vi "util_timer.vi"(7 "timer_command":T2=enum."read", 8 "error in (no error)":errorcluster, 10 "current_time":dbl=nan format="%#_13g", 11 "timer in":T1 {"previous_time" format="%<%H:%M:%S%3u>t"; "elapsed_time" format="%<%H:%M:%S%3u>t"}) -> (0 "error out":errorcluster, 2 "elapsed_time":dbl format="%#_13g", 3 "timer out":T1 {"previous_time" format="%<%H:%M:%S%3u>t"; "elapsed_time" format="%<%H:%M:%S%3u>t"})   [LabVIEW 2015, in "lv-recipe-machine.lvlib"]
uses:
  lv-recipe-machine.lvlib
  _controls/timer_command.ctl
  public/_controls/timer.ctl
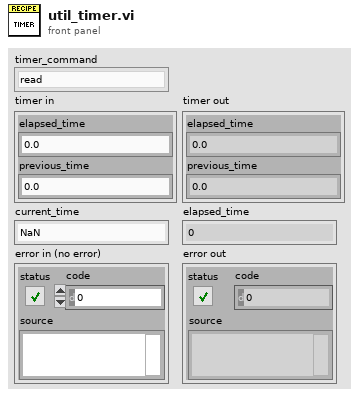
[diagram p1: front panel]
types:
  T1 = typedef "lv-recipe-machine.lvlib/timer.ctl" = cluster{"elapsed_time":dbl, "previous_time":dbl}
  T2 = typedef "lv-recipe-machine.lvlib/timer_command.ctl" = enum16{"<timer_command>", "start", "read", "pause", "resume", "stop", "<null>"}
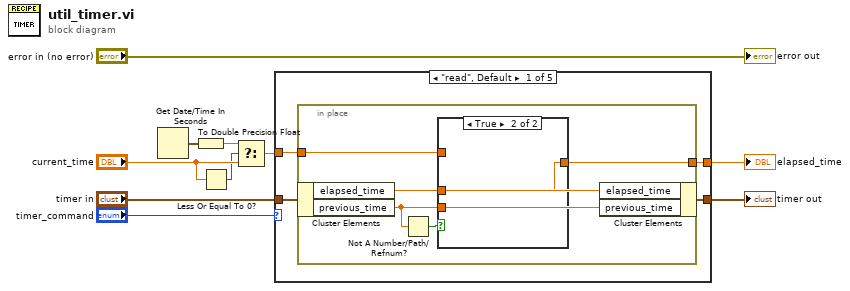
[diagram p0: block diagram]
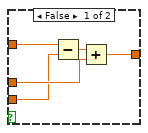
[diagram p2: hidden frame]
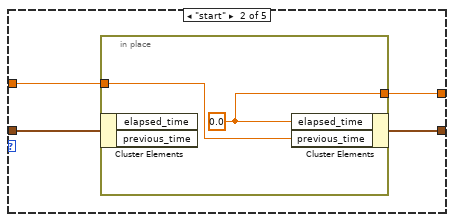
[diagram p3: hidden frame]
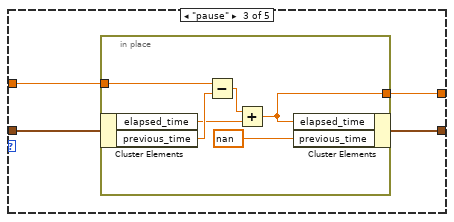
[diagram p4: hidden frame]
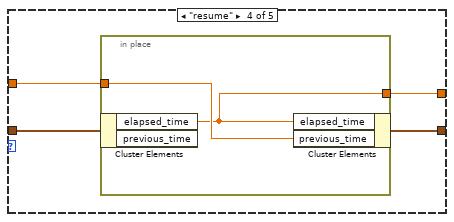
[diagram p5: hidden frame]
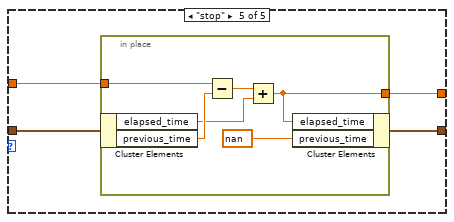
[diagram p6: hidden frame]
diagram:
  n1 = Get Date/Time In Seconds() -> (seconds since 1Jan1904=w3:timestamp)
  n2 = To Double Precision Float(number=w3) -> (double precision float=w2:dbl)
  n3 = Less Or Equal To 0?(x="current_time") -> (x <= 0?=w4:bool)
  n4 = Select(t=w2, s=w4, f="current_time") -> (s? t:f=w1:dbl)
  n5 = case shown="\"read\", Default" "timer_command" {
    tunnel: "timer in" -> [w14 w29 w35 w45 w51]
    tunnel: w1 -> [w13 w28 w34 w44 w50]
    tunnel: [w12 w27 w33 w43 w49] -> w6
    tunnel: [w11 w26 w32 w42 w48] -> w5
    frame "read", Default {
      n6 = in-place {
        in-place-border: w13 -> [w19]
        in-place-border: [w17] -> w11
        n7 = in-place-cluster #1(w14) -> ("elapsed_time"=w18:dbl, "previous_time"=w16:dbl)
        n8 = Not A Number/Path/Refnum?(number/path/refnum=w16) -> (NaN/Path/Refnum?=w15:bool)
        n9 = case shown="True" w15 {
          tunnel: w19 -> [w24 _]
          tunnel: w18 -> [w23 w25]
          tunnel: w16 -> [w22 _]
          tunnel: [w20 w25] -> w17
          frame False {
            n10 = Subtract(x=w24, y=w22) -> (x-y=w21:dbl)
            n11 = Add(x=w21, y=w23) -> (x+y=w20:dbl)
          }
          frame True {
          }
        }
        n12 = in-place-cluster #1("elapsed_time"=w18, "previous_time"=w16) -> (w12:T1)
      }
    }
    frame "start" {
      n13 = in-place {
        in-place-border: w28 -> [w31]
        in-place-border: [w30] -> w26
        w30 = 0.0 ("elapsed_timer")
        n14 = in-place-cluster #2(w29) -> ()  [unwired: 2 out]
        n15 = in-place-cluster #2("elapsed_time"=w30, "previous_time"=w31) -> (w27:T1)
      }
    }
    frame "pause" {
      n16 = in-place {
        in-place-border: w34 -> [w41]
        in-place-border: [w36] -> w32
        n17 = in-place-cluster #3(w35) -> ("elapsed_time"=w38:dbl, "previous_time"=w40:dbl)
        n18 = Subtract(x=w41, y=w40) -> (x-y=w39:dbl)
        n19 = Add(x=w39, y=w38) -> (x+y=w36:dbl)
        n20 = in-place-cluster #3("elapsed_time"=w36, "previous_time"=nan) -> (w33:T1)
      }
    }
    frame "resume" {
      n21 = in-place {
        in-place-border: w44 -> [w47]
        in-place-border: [w46] -> w42
        n22 = in-place-cluster #4(w45) -> ("elapsed_time"=w46:dbl)  [unwired: 1 out]
        n23 = in-place-cluster #4("elapsed_time"=w46, "previous_time"=w47) -> (w43:T1)
      }
    }
    frame "stop" {
      n24 = in-place {
        in-place-border: w50 -> [w56]
        in-place-border: [w52] -> w48
        n25 = in-place-cluster #5(w51) -> ("elapsed_time"=w54:dbl, "previous_time"=w55:dbl)
        n26 = Subtract(x=w56, y=w55) -> (x-y=w53:dbl)
        n27 = Add(x=w53, y=w54) -> (x+y=w52:dbl)
        n28 = in-place-cluster #5("elapsed_time"=w52, "previous_time"=nan ("elapsed_timer")) -> (w49:T1)
      }
    }
  }
  "timer out" <- w6
  "elapsed_time" <- w5
  "error out" <- "error in (no error)"
